vi "Read Test Method Count.vi"(11 "Test Suite Result In":refnum<class "Test Suite Result.lvclass">) -> (1 "Test Method count string":string, 2 "Test Method count":i32, 3 "Test Suite Result Out":refnum<class "Test Suite Result.lvclass">)   [LabVIEW 2020, in "Test Suite Result.lvclass"]
uses:
  Test Suite Result.lvclass
  Test Suite Result.lvclass/Test Suite Result.ctl
  Test Case Result/Test Case Result.lvclass/Test Case Result.ctl
  Test Case Result/Test Case Result.lvclass
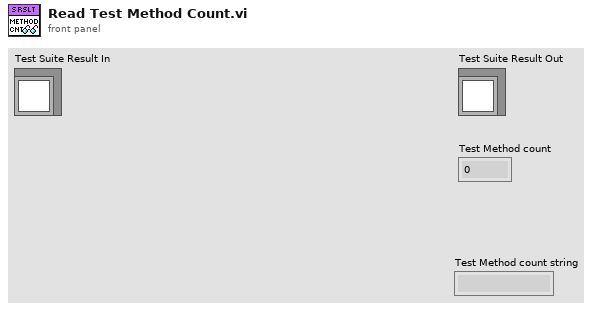
[diagram p1: front panel]
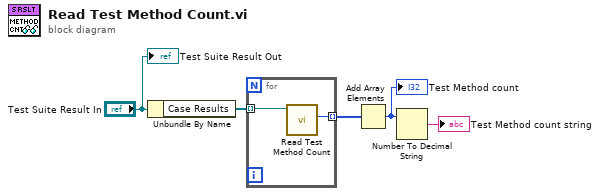
[diagram p0: block diagram]
diagram:
  n1 = Unbundle By Name("Test Suite Result In") -> ("Case Results"=w3:refnum<class "Test Case Result.lvclass">[])
  n2 = for {
    tunnel: w3 -> [w7] mode=indexing
    tunnel: [w6] -> w2 mode=indexing
    n3 = call "Read Test Method Count.vi"("Test Case Result In"=w7) -> ("Numeric"=w6:i32)  [unwired: 9 in, 1 out]
  }
  n4 = Add Array Elements(numeric array=w2) -> (sum=w1:i32)
  "Test Method count" <- w1
  n5 = Number To Decimal String(number=w1) -> (decimal integer string=→"Test Method count string":string)  [unwired: 1 in]
  "Test Suite Result Out" <- "Test Suite Result In"
